vi "Calc Lift Speeds.vi"(9 "Lift Speed":dbl) -> (3 "Lift Speed":dbl)   [LabVIEW 2019]
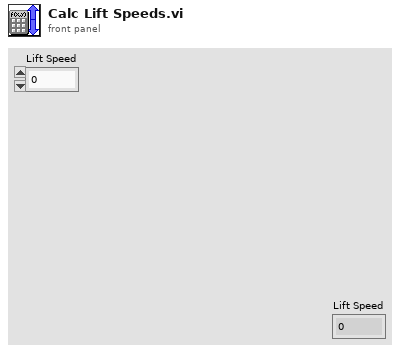
[diagram p1: front panel]
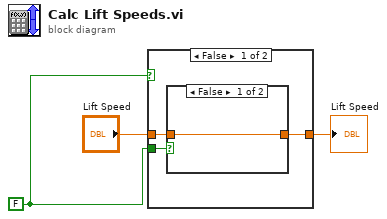
[diagram p0: block diagram]
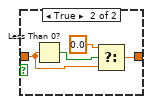
[diagram p2: hidden frame]
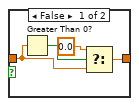
[diagram p4: hidden frame]
diagram:
  w1 = FALSE
  n1 = case shown="False" w1 {
    tunnel: "Lift Speed" -> [w6 w14]
    tunnel: [w5 w13] -> w3
    tunnel: w1 -> [w4 w12]
    frame False {
      n2 = case shown="False" w4 {
        tunnel: w6 -> [w7 w9]
        tunnel: [w7 w8] -> w5
        frame False {
        }
        frame True {
          n3 = Less Than 0?(x=w9) -> (x < 0?=w11:bool)
          n4 = Select(t=0.0, s=w11, f=w9) -> (s? t:f=w8:dbl)
        }
      }
    }
    frame True {
      n5 = case shown="True" w12 {
        tunnel: w14 -> [w16 w19]
        tunnel: [w15 w19] -> w13
        frame False {
          n6 = Greater Than 0?(x=w16) -> (x > 0?=w18:bool)
          n7 = Select(t=0.0, s=w18, f=w16) -> (s? t:f=w15:dbl)
        }
        frame True {
        }
      }
    }
  }
  "Lift Speed" <- w3
